vi "Update Public Data.vi"(2 "Variant In":variant, 3 "Public 2":refnum<vi>) -> (0 "Variant Out":variant, 1 "Public":T1)   [LabVIEW 2021]
uses:
  Sub Controls/Public.ctl
panel:
  out "error out":errorcluster
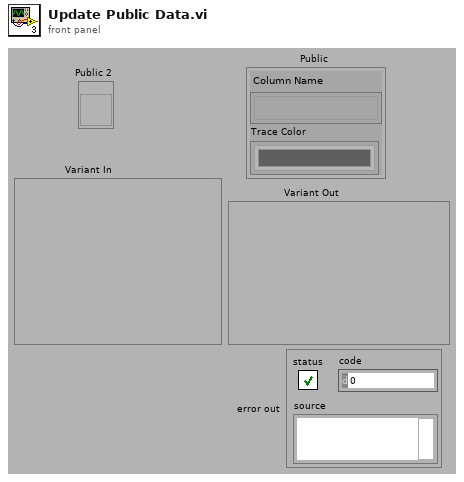
[diagram p1: front panel]
types:
  T1 = typedef "Public.ctl" = cluster{"Column Name":string[], "Trace Color":u32[]}
  T2 = typedef "Instrument Properties.ctl" = cluster{"Public":T1, "Private":T3}
  T3 = typedef "Private.ctl" = cluster{"Path":path, "VI Refnum":T4, "Name":string, "# of Values":i32, "Scale Factors":dbl[], "Display":T5[], "Offset":dbl[]}
  T4 = typedef "Instrument Ref.ctl" = refnum<vi>
  T5 = typedef "SystemCheckBox-resize.ctl" = bool
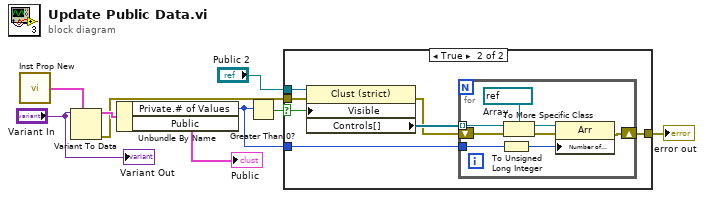
[diagram p0: block diagram]
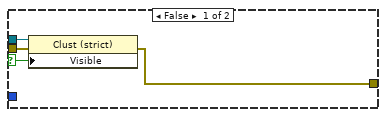
[diagram p2: hidden frame]
diagram:
  n1 = call "Inst Prop New.vi"() -> ("Instrument Prop Out"=w9:T2)
  n2 = Variant To Data(type=w9, Variant="Variant In") -> (data=w8:T2, error out=w2:errorcluster)  [unwired: 1 in]
  n3 = Unbundle By Name(w8) -> ("Private.# of Values"=w5:i32, "Public"=→"Public":T1)
  n4 = Greater Than 0?(x=w5) -> (x > 0?=w4:bool)
  n5 = case shown="True" w4 {
    selector: w4 -> [w12 w19]
    tunnel: "Public 2" -> [w13 w20]
    tunnel: w5 -> [_ w17]
    tunnel: w2 -> [w11 w16]
    tunnel: [w10 w14] -> w1
    frame False {
      n6 = property class="Clust (strict)"(reference=w13, error in=w11, "Visible"=w12) -> (error out=w10:errorcluster)  [unwired: 1 out]
    }
    frame True {
      n7 = property class="Clust (strict)"(reference=w20, error in=w16, "Visible"=w19) -> (error out=w15:errorcluster, "Controls[]"=w18:refnum<vi>[])  [unwired: 1 out]
      n8 = for {
        tunnel: w18 -> [w28] mode=indexing
        tunnel: w17 -> [w25]
        shift-right: [w21] -> w14
        shift-left: w15 -> [w23]
        w26 = refnum<vi> refnum  # Array
        n9 = To Unsigned Long Integer(number=w25) -> (unsigned 32bit integer=w24:u32)
        n10 = To More Specific Class(target class=w26, reference=w28, error in=w23) -> (specific class reference=w27:refnum<vi>, error out=w22:errorcluster)
        n11 = property class="Arr"(reference=w27, error in=w22, "Number of Columns"=w24) -> (error out=w21:errorcluster)  [unwired: 1 out]
      }
    }
  }
  "error out" <- w1
  "Variant Out" <- "Variant In"
